vi "题目4.vi"() -> ()   [LabVIEW 2017]
uses:
  <vilib>/measure/NI_MABase.lvlib
panel:
  out "大小":i32
  out "Y":dbl[](array[numeric])
  out "最小值":dbl
  out "dt":dbl
  out "signal out":waveform(dbl) caption="信号输出"
  out "error out":errorcluster caption="错误输出"
  in  "frequency":dbl=10.0 caption="频率" format="%.2p"
  in  "amplitude":dbl=1.0 caption="幅值" format="%.2p"
  in  "phase":dbl caption="相位" format="%.2p"
  in  "error in (no error)":errorcluster caption="错误输入（无错误）"
  in  "reset signal":bool caption="重置信号"
  in  "sampling info":cluster{"Fs":dbl, "#s":dbl}={"Fs"=1000.0, "#s"=1000.0} caption="采样信息" {"Fs" format="%.2p"}
  in  "offset":dbl caption="偏移量" format="%.2p"
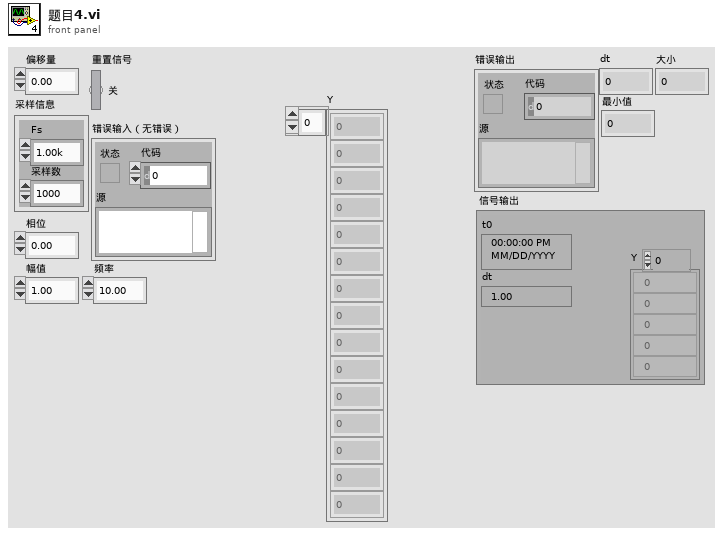
[diagram p1: front panel]
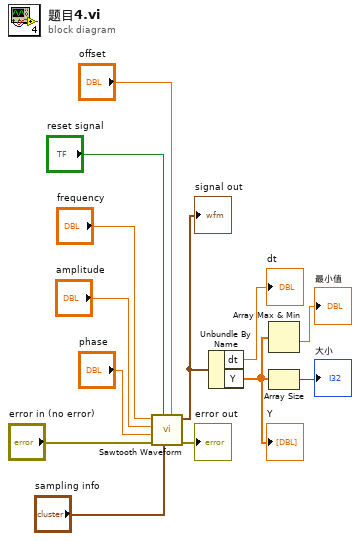
[diagram p0: block diagram]
diagram:
  n1 = call <vilib>:"Sawtooth Waveform.vi"("offset"="offset", "sampling info"="sampling info", "reset signal"="reset signal", "error in (no error)"="error in (no error)", "phase"="phase", "amplitude"="amplitude", "frequency"="frequency") -> ("error out"=→"error out":errorcluster, "signal out"=w5:waveform(dbl))  [unwired: 3 in]
  "signal out" <- w5
  n2 = Unbundle By Name(w5) -> ("dt"=→"dt":dbl, "Y"=w1:dbl[])
  "Y" <- w1
  n3 = Array Max & Min(array=w1) -> (min value=→"最小值":dbl)  [unwired: 3 out]
  n4 = Array Size(array=w1) -> (size(s)=→"大小":i32)
